vi "Main.vi"() -> ()   [LabVIEW 2014]
uses:
  <vilib>/Analysis/2dsp.llb/Real FFT.vi
  <vilib>/Analysis/5stat.llb/RMS (DBL).vi
  <vilib>/Analysis/2dsp.llb/Inverse Real FFT.vi
  <vilib>/gmath/NI_Gmath.lvlib
  <vilib>/Analysis/NI_AALPro.lvlib
panel:
  out "controlling rms value":dbl format="%0.2f"
  out "Shifted FFT":dbl[](graph)
  out "Input FFT":dbl[](graph)
  out "Output":waveform(dbl)(graph) caption="Output Note"
  out "input rms value":dbl format="%0.2f"
  out "freq ratio":dbl
  out "main timbre freq":dbl
  out "control freq":dbl format="%.2f"
  in  "stop":bool caption="freq control"
  out "Controlling Note":dynamicdata(graph)
  out "Input Note":dynamicdata(graph)
  in  "timbre (F)":bool caption="timbre record"
  # "Records one sample length (about one second).  For the timbre record."
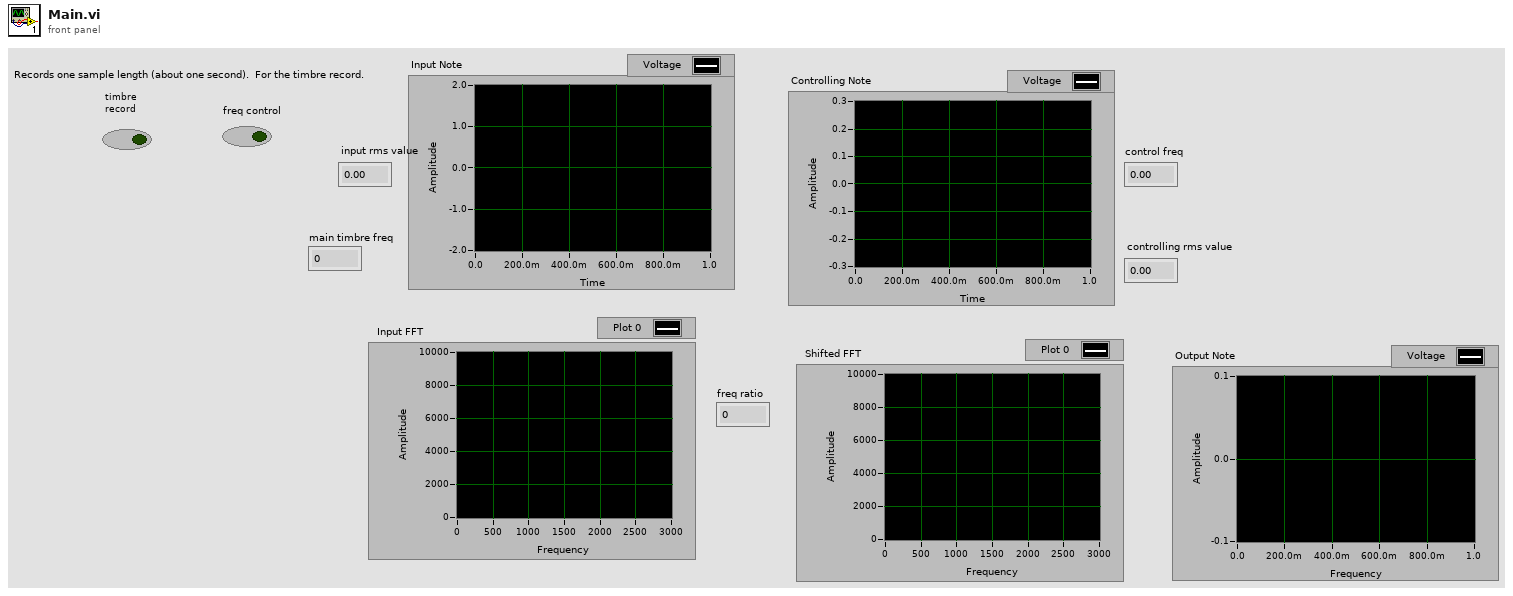
[diagram p1: front panel]
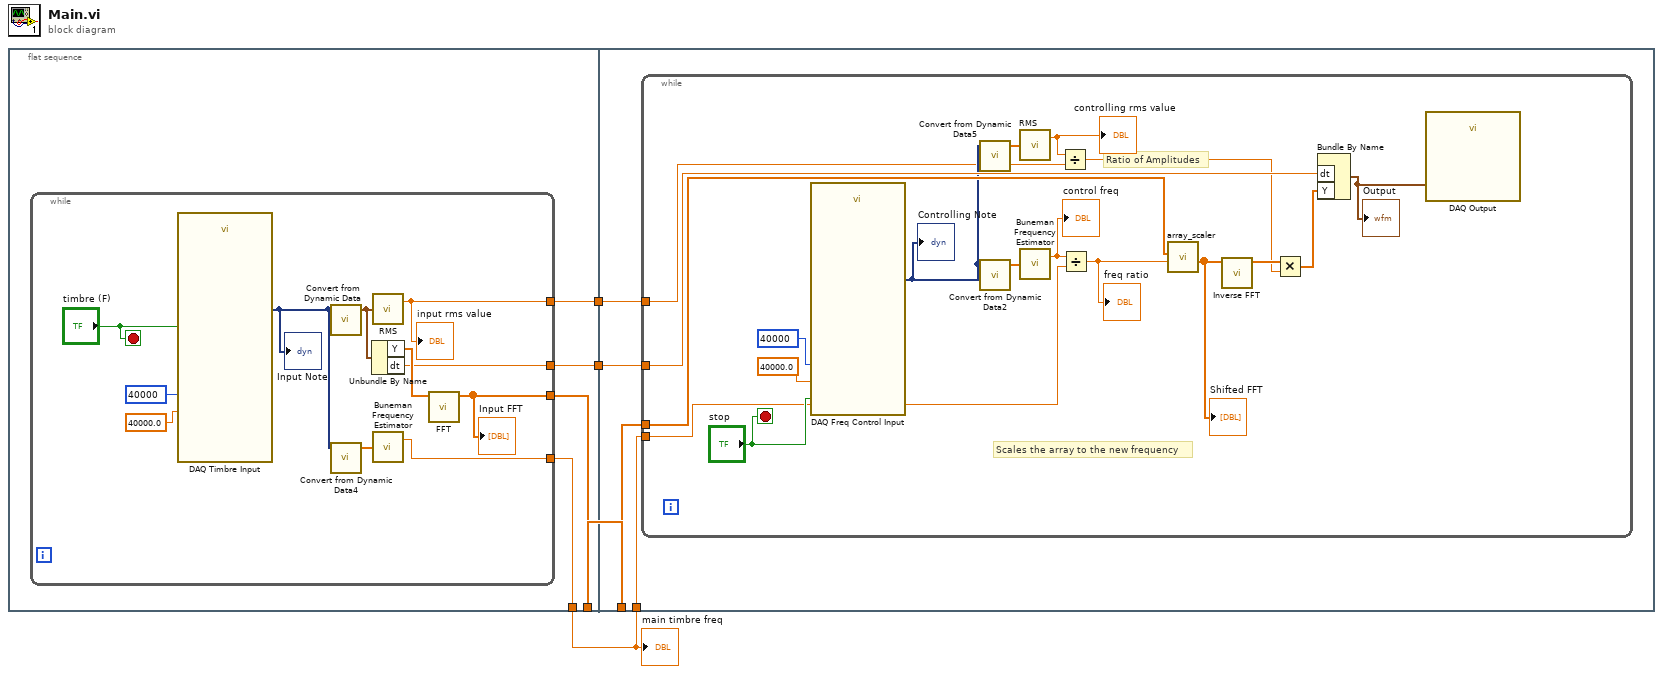
[diagram p0: block diagram]
diagram:
  n1 = flat-sequence {
    tunnel: [w8] -> w4
    tunnel: [w7] -> w3
    tunnel: [w6] -> w2
    tunnel: [w5] -> w1
    tunnel: w4 -> [w23]
    tunnel: w3 -> [w22]
    tunnel: w2 -> [w21]
    tunnel: w1 -> [w20]
    frame #0 {
      n2 = while {
        tunnel: [w15] -> w8
        tunnel: [w10] -> w7
        tunnel: [w12] -> w6
        tunnel: [w11] -> w5
        stop <- "timbre (F)" stop-if-true
        n3 = call "DAQ Timbre Input"("rate"=40000.0, "number of samples"=40000, "stop (T)"="timbre (F)") -> ("data"=w9:dynamicdata)  [unwired: 14 in, 2 out]
        "Input Note" <- w9
        n4 = call "Convert from Dynamic Data"("Dynamic Data Type"=w9) -> ("Waveform"=w14:waveform(dbl))  [unwired: 3 in]
        n5 = call "Convert from Dynamic Data4"("Dynamic Data Type"=w9) -> ("Array"=w16:dbl[])  [unwired: 3 in]
        n6 = Unbundle By Name(w14) -> ("Y"=w13:dbl[], "dt"=w12:dbl)
        n7 = call-poly <vilib>:"RMS.vi"("X"=w14) -> ("rms value"=w11:dbl)  [unwired: 1 out]
        "input rms value" <- w11
        n8 = call <vilib>:"Buneman Frequency Estimator.vi"("X"=w16) -> ("beta"=w15:dbl)  [unwired: 1 out]
        n9 = call-poly <vilib>:"FFT.vi"("X"=w13) -> ("FFT {X}"=w10:cdb[])  [unwired: 9 in, 1 out]
        "Input FFT" <- w10
      }
    }
    frame #1 {
      n10 = while {
        tunnel: w23 -> [w38]
        tunnel: w22 -> [w34]
        tunnel: w21 -> [w35]
        tunnel: w20 -> [w28]
        stop <- "stop" stop-if-true
        # "Scales the array to the new frequency"
        # "Ratio of Amplitudes"
        n11 = call "DAQ Freq Control Input"("rate"=40000.0, "number of samples"=40000, "stop (T)"="stop") -> ("data"=w31:dynamicdata)  [unwired: 14 in, 2 out]
        "Controlling Note" <- w31
        n12 = call "Convert from Dynamic Data5"("Dynamic Data Type"=w31) -> ("Array"=w30:dbl[])  [unwired: 3 in]
        n13 = call "Convert from Dynamic Data2"("Dynamic Data Type"=w31) -> ("Array"=w41:dbl[])  [unwired: 3 in]
        n14 = call-poly <vilib>:"RMS.vi"("X"=w30) -> ("rms value"=w29:dbl)  [unwired: 1 out]
        "controlling rms value" <- w29
        n15 = call <vilib>:"Buneman Frequency Estimator.vi"("X"=w41) -> ("beta"=w39:dbl)  [unwired: 1 out]
        "control freq" <- w39
        n16 = Divide(x=w29, y=w28) -> (x/y=w25:dbl)
        n17 = Divide(x=w39, y=w38) -> (x/y=w27:dbl)
        "freq ratio" <- w27
        n18 = call "array_scaler.vi"("array"=w34, "scale"=w27) -> ("output array"=w26:dbl[])  [unwired: 8 in]
        "Shifted FFT" <- w26
        n19 = call-poly <vilib>:"Inverse FFT.vi"("FFT {X}"=w26) -> ("X"=w33:dbl[])  [unwired: 9 in, 1 out]
        n20 = Multiply(x=w33, y=w25) -> (x*y=w32:dbl[])
        n21 = Bundle By Name("dt"=w35, "Y"=w32) -> (w24:waveform(dbl))  [unwired: 1 in]
        "Output" <- w24
        n22 = call "DAQ Output"("data"=w24) -> ()  [unwired: 17 in, 2 out]
      }
    }
  }
  "main timbre freq" <- w4
